vi "path.vi"(1 "file":string, 2 "path_in":path) -> (0 "path_out":string)   [LabVIEW 2012]
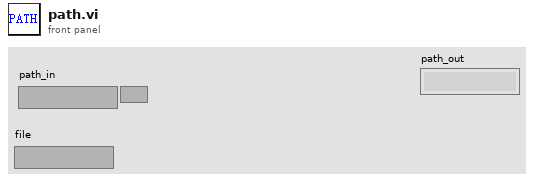
[diagram p1: front panel]
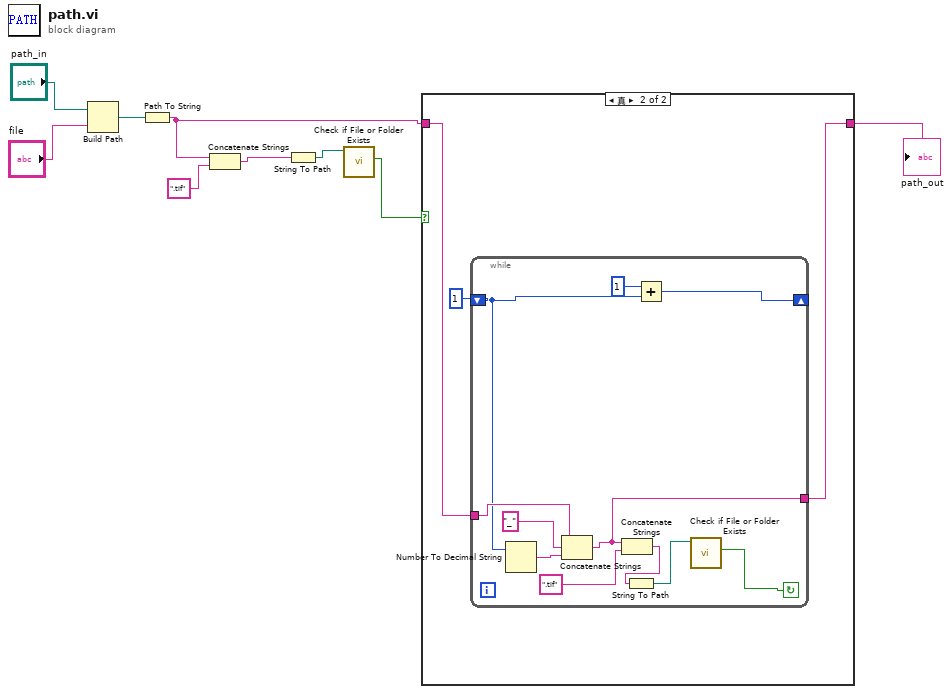
[diagram p0: block diagram]
diagram:
  n1 = Build Path(base path="path_in", name or relative path="file") -> (appended path=w7:path)
  n2 = Path To String(path=w7) -> (string=w2:string)
  n3 = Concatenate Strings(w2, ".tif" ("字符串")) -> (w5:string)
  n4 = String To Path(string=w5) -> (path=w4:path)
  n5 = call <vilib>:"Check if File or Folder Exists.vi"("path"=w4) -> ("file or folder exists?"=w3:bool)  [unwired: 8 in, 2 out]
  n6 = case shown="真" w3 {
    tunnel: w2 -> [w10 w12]
    tunnel: [w10 w11] -> w1
    frame False {
    }
    frame True {
      n7 = while {
        shift-right: [w23] -> _
        shift-left: 1 -> [w21]
        tunnel: w12 -> [w22]
        tunnel: [w14] -> w11
        stop <- w17 continue-if-true
        n8 = Number To Decimal String(number=w21) -> (decimal integer string=w20:string)  [unwired: 1 in]
        n9 = Concatenate Strings(w22, "_" ("字符串"), w20) -> (w14:string)
        n10 = Concatenate Strings(w14, ".tif" ("字符串")) -> (w15:string)
        n11 = String To Path(string=w15) -> (path=w18:path)
        n12 = Add(x=1, y=w21) -> (x+y=w23:i32)
        n13 = call <vilib>:"Check if File or Folder Exists.vi"("path"=w18) -> ("file or folder exists?"=w17:bool)  [unwired: 8 in, 2 out]
      }
    }
  }
  "path_out" <- w1
